vi "CgtpPauseAllPrograms.vi"(10 "Cgtp":refnum<k24>, 11 "error in":errorcluster) -> (3 "error out":errorcluster)   [LabVIEW 2011, in "UnderAutomation.Fanuc.lvlib"]
uses:
  UnderAutomation.Fanuc.lvlib
  C:/Users/fg/Documents/Fanuc.vi/LabVIEW_2024/UnderAutomation.Fanuc/lib/UnderAutomation.Fanuc.dll
  LabVIEW_2024/UnderAutomation.Fanuc/lib/UnderAutomation.Fanuc.dll
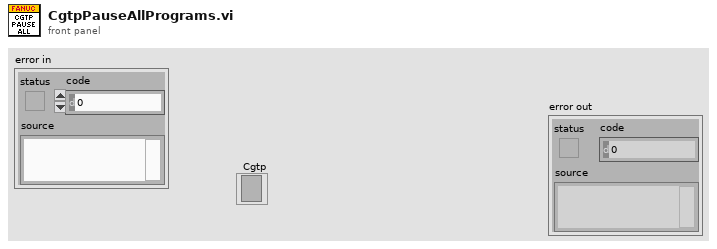
[diagram p1: front panel]
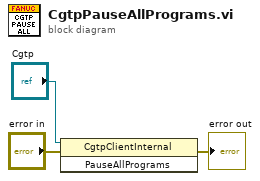
[diagram p0: block diagram]
diagram:
  n1 = invoke class="CgtpClientInternal" method="PauseAllPrograms"(reference="Cgtp", error in="error in") -> (error out=→"error out":errorcluster)  [unwired: 1 in, 2 out]
